vi "PGPASS default path.vi"(8 "error in (no error)":errorcluster) -> (0 "error out":errorcluster, 3 "PGPASS path":path)   [LabVIEW 2016, in "PQ Support.lvlib"]
uses:
  PQ Support.lvlib
  <vilib>/Utility/sysdir.llb/System Directory Type.ctl
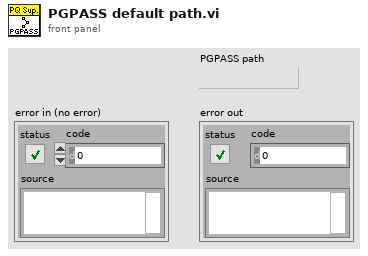
[diagram p1: front panel]
types:
  T1 = typedef "System Directory Type.ctl" = i32
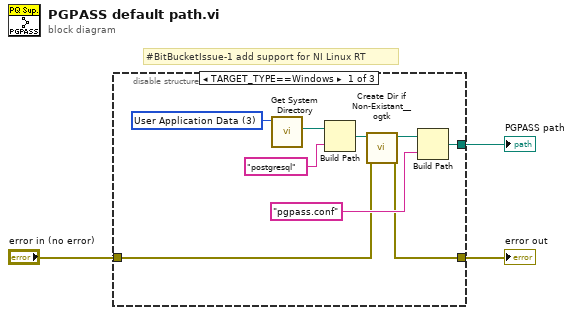
[diagram p0: block diagram]
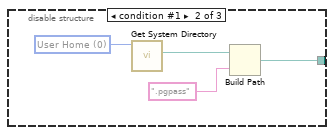
[diagram p2: hidden frame]
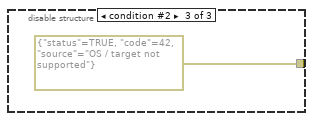
[diagram p3: hidden frame]
diagram:
  # "#BitBucketIssue-1 add support for NI Linux RT"
  n1 = disable-structure shown="TARGET_TYPE==Windows" {
    disable-tunnel: [w8 w13 _] -> w1
    disable-tunnel: [w4 _ errorcluster {"status"=TRUE, "code"=42, "source"="OS / target not supported"} ("error in (no error)")] -> w2
    disable-tunnel: "error in (no error)" -> [w5 _ _]
    frame condition #0 (active) {
      w12 = T1 3 items=["User Home"=0, "User Desktop"=1, "User Documents"=2, "User Application Data"=3, "User Preferences"=4, "User Temporary"=5, "Public Documents"=6, "Public Application Data"=7, "Public Preferences"=8, "Public Cache"=13, "System Core Libraries"=9, "System Installed Libraries"=10, "Application Files"=11, "Boot Volume Root"=12] ("system directory type")
      n2 = call <vilib>:"Get System Directory.vi"("system directory type"=w12) -> ("system directory"=w11:path)  [unwired: 10 in]
      n3 = Build Path(base path=w11, name or relative path="postgresql") -> (appended path=w7:path)
      n4 = call <userlib>:"Create Dir if Non-Existant__ogtk.vi"("error in (no error)"=w5, "Directory Path"=w7) -> ("error out"=w4:errorcluster, "dup Directory Path"=w6:path)  [unwired: 7 in, 1 out]
      n5 = Build Path(base path=w6, name or relative path="pgpass.conf") -> (appended path=w8:path)
    }
    frame condition #1 {
      w16 = T1 0 items=["User Home"=0, "User Desktop"=1, "User Documents"=2, "User Application Data"=3, "User Preferences"=4, "User Temporary"=5, "Public Documents"=6, "Public Application Data"=7, "Public Preferences"=8, "Public Cache"=13, "System Core Libraries"=9, "System Installed Libraries"=10, "Application Files"=11, "Boot Volume Root"=12] ("system directory type")
      n6 = call <vilib>:"Get System Directory.vi"("system directory type"=w16) -> ("system directory"=w14:path)  [unwired: 10 in]
      n7 = Build Path(base path=w14, name or relative path=".pgpass") -> (appended path=w13:path)
    }
    frame condition #2 {
    }
  }
  "error out" <- w2
  "PGPASS path" <- w1
